vi "Dashboard Main.vi"() -> ()   [LabVIEW 2017]
uses:
  <vilib>/Rock Robotics/WPI/DriverStation/WPI_DriverStationAllianceInfo.ctl
  <vilib>/Rock Robotics/WPI/DriverStation/WPI_DriverStationPositionInfo.ctl
  <vilib>/Utility/miscctls.llb/LVRowAndColumnTypeDef.ctl
  <vilib>/event_ctls.llb/eventvkey.ctl
  <vilib>/Rock Robotics/Network Tables/NT Read Numeric Array.vi
  <vilib>/Rock Robotics/Network Tables/NT Write String Array.vi
  <vilib>/Rock Robotics/Network Tables/NT Write Numeric Array.vi
  <vilib>/Rock Robotics/Network Tables/NT Write Boolean.vi
  <vilib>/Rock Robotics/WPI/Dashboard/WPI_DashboardLogging Global.vi
panel:
  in  "Camera Settings Right":T1={"Frame Rate"=30, "Compression"=30, "Size"=1, "DB Camera Config"=FALSE} {"Frame Rate" scale=1.0..30.0; "Compression" scale=100.0..-1.0; "Size" items=["640x480", "320x240", "160x120"]}
  in  "Camera Name Right":string(combo)="No Camera Selection"
  out "Camera Info":cluster{"Mbps LED":bool, "Mbps":dbl, "fps":dbl} {"fps" format="%#.1g"; "Mbps" format="%#.1g"}
  in  "Camera Settings":T1={"Frame Rate"=30, "Compression"=30, "Size"=1, "DB Camera Config"=FALSE} {"Frame Rate" scale=1.0..30.0; "Compression" scale=100.0..-1.0; "Size" items=["640x480", "320x240", "160x120"]}
  in  "TCP":refnum<k5>
  in  "Rec Mode":enum32{"Stop", "Record", "Playback"}(radio)
  out "Robot IP":string
  out "Image Message":string="Timeout in Camera Communications"
  in  "Dashboard Tab":T2(tab)
  in  "Scooter Scale":dbl(slide)=0.49999999999999994 scale=0.0..1.0
  in  "Select Auto":string(combo)="Select Autonomous ..."
  out "NT Connection":bool
  out "MotorChart R":cluster{"Numeric":dbl, "Numeric":dbl}(graph)
  out "MotorChart L":cluster{"Numeric":dbl, "Numeric":dbl}(graph)
  out "MotorSliders R":cluster{"MotorSlide1":dbl, "MotorSlide2":dbl} {"MotorSlide2" scale=-1.0..1.0 scale format="%#_2e"; "MotorSlide1" scale=-1.0..1.0 scale format="%#_2e"}
  out "MotorSliders L":cluster{"MotorSlide1":dbl, "MotorSlide2":dbl} {"MotorSlide2" scale=-1.0..1.0 scale format="%#_2e"; "MotorSlide1" scale=-1.0..1.0 scale format="%#_2e"}
  out "Gyro":dbl(knob) scale=0.0..360.0
  out "JS1 Z":dbl(slide) scale=-1.0..1.0 scale format="%#_2e"
  out "JS1 Graph":cluster{"X":dbl, "Y":dbl}[](graph)
  out "JS1 Buttons":T3
  out "JS2 Z":dbl(slide) scale=-1.0..1.0 scale format="%#_2e"
  out "JS2 Graph":cluster{"X":dbl, "Y":dbl}[](graph)
  out "JS2 Buttons":T3
  out "Mode":T4(ring)=enum."Auto Disabled"
  out "Vision Angle":dbl
  out "Robot IP 2":string
  in  "Scooter Button":bool
  in  "Invert Drive?":bool
  out "Camera Image Right":T5(plugin-control)
  in  "DB/String 9":string
  in  "DB/String 8":string
  in  "DB/String 7":string
  in  "DB/String 6":string
  in  "DB/String 5":string
  in  "DB/String 4":string
  in  "DB/String 3":string
  in  "DB/String 2":string
  in  "DB/String 1":string
  in  "DB/String 0":string
  in  "DB/Slider 0":dbl(slide) scale=0.0..5.0
  in  "DB/Slider 1":dbl(slide) scale=0.0..5.0
  in  "DB/Slider 2":dbl(slide) scale=0.0..5.0
  in  "DB/Slider 3":dbl(slide) scale=0.0..5.0
  out "DB/LED 3":bool
  out "DB/LED 2":bool
  out "DB/LED 1":bool
  out "DB/LED 0":bool
  in  "DB/Button 3":bool
  in  "DB/Button 2":bool
  in  "DB/Button 1":bool
  in  "DB/Button 0":bool caption="New Name"
  out "Motor Outputs":T6 {"Motor 7" scale=-1.0..1.0; "Motor 6" scale=-1.0..1.0; "Motor 5" scale=-1.0..1.0; "Motor 4" scale=-1.0..1.0; "Motor 3" scale=-1.0..1.0; "Motor 2" scale=-1.0..1.0; "Motor 1" scale=-1.0..1.0; "Motor 0" scale=-1.0..1.0}
  out "Encoder Data":dbl[](array[numeric])
  out "NavX Data":dbl[](array[numeric])
  in  "Test Slider":dbl(slide) scale=0.0..100.0 scale format="%#_3g"
  in  "On/Off":bool caption="Solenoid"
  in  "Test Name":u16(ring) items=["Select the test to run..."]
  in  "Test Tree":string(tree)
  in  "Motor":cluster{"Value":dbl, "Enable":bool} {"Value" scale=-1.0..1.0 scale format="%#_3g"}
  out "Progress":T7 {"Test Progress" scale=0.0..100.0}
  in  "Rev/Fwd":cluster{"Forward":bool, "Reverse":bool}
  in  "Test Ring":u16(ring) items=["Monochrome", "Color"]
  out "Cmd Status":string
  in  "Execute Command":bool
  in  "Command Params":string[][](table)
  in  "Command Selection":i32(listbox)
  in  "CheckList":i32(listbox)
  out "Tree":string(tree)
  in  "Debug Data 2":dbl[](array[numeric])
  in  "Vision Target Offset":dbl=2.5
  in  "Vision Target Angle":dbl=15.0
  in  "Jog Mode Refnum":string(combo)="frontLeftRotation"
  out "Match Time":dbl
  in  "Debug Data":dbl[](array[numeric])
  in  "Debug Commands":string[](array[combo])
  in  "Debug Command?":bool
  out "Command Data":dbl[](array[numeric])
  out "Output Commands":string[](array[string])
  out "30 Amp Plugs":dbl[](array[slide]) scale=0.0..30.0
  out "40 Amp Plugs":dbl[](array[slide]) scale=0.0..40.0
  out "Ultrasonic Distance":dbl
  in  "Shooter Speed":dbl=0.575
  in  "Alliance":T8
  in  "Position":T9
  out "Command Data 2":dbl[](array[numeric])
  out "Camera Image":T5(plugin-control)
  out "Background":bool
  in  "Camera Name":string(combo)="No Camera Selection"
  # "HW"
  # "HW"
  # "Joysticks"
  # "Joystick 0 Layout\nAlign Left Gear: X\nAlign Middle Gear: A\nAlign Right Gear: B\nDrive To Shot Dist: Y\nVision Align: Left Bumper\nGear Place: Right Bumper\nBack: Command Stop\nStart: Reset Gyro\nR3: Jog Mode (Axis 1)\n\nJoystick 1 Layout\nShooter Forwards: Y\nShooter Backwards: A\nLift Up: B\nLift Down: Start\nLift Override Up: Back\nIntake In: Left Bumper\nIntake Out: Right Bumper\nAgitator In: D-Pad Up\nAgitator Out: D-Pad Down"
  # "Drive Motors"
  # "Front"
  # "Right"
  # "Left"
  # "Back"
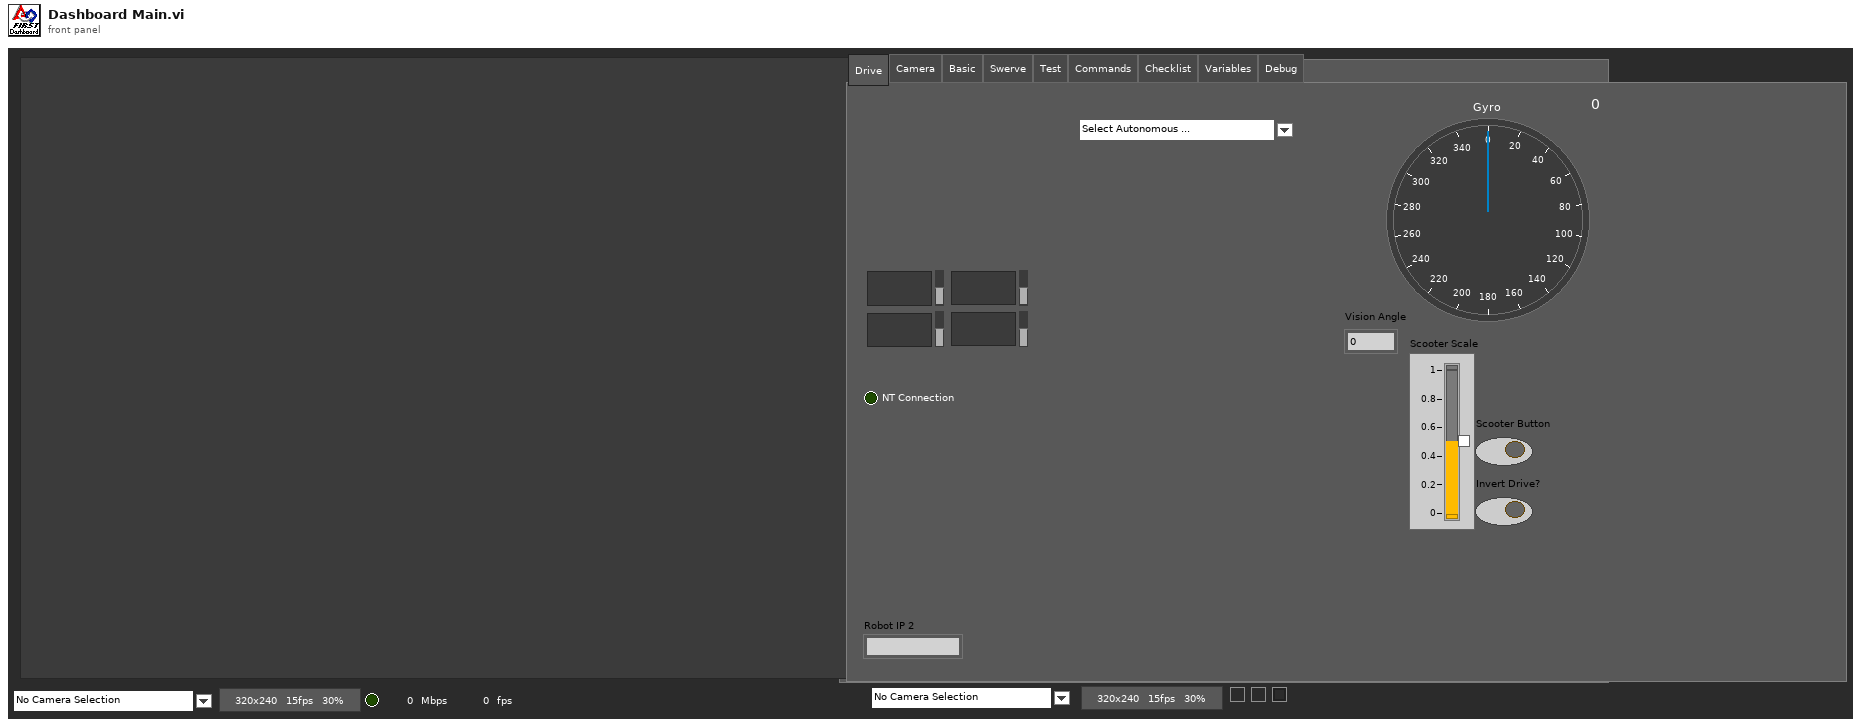
[diagram p1: front panel]
types:
  T1 = cluster{"Frame Rate":i32, "Compression":i32, "Size":u16, "DB Camera Config":bool}
  T2 = enum32{"Drive", "Camera", "Basic", "Swerve", "Test", "Commands", "Checklist", "Variables", "Debug"}
  T3 = cluster{bool, bool, bool, bool, bool, bool, bool, bool, bool, bool, bool, bool}
  T4 = enum8{"Tele-Op Disabled", "Tele-Op Enabled", "Auto Disabled", "Auto Enabled", "Test Disabled", "Test Enabled", "Disconnected", "No Code", "E-Stop"}
  T5 = typedef "IMAQ Image.ctl" = refnum<image>
  T6 = cluster{"Motor 0":dbl, "Motor 1":dbl, "Motor 2":dbl, "Motor 3":dbl, "Motor 4":dbl, "Motor 5":dbl, "Motor 6":dbl, "Motor 7":dbl}
  T7 = cluster{"Test Progress":u8, "Test Progress Text":string}
  T8 = typedef "WPI_DriverStationAllianceInfo.ctl" = enum16{"Red", "Blue", "Invalid"}
  T9 = typedef "WPI_DriverStationPositionInfo.ctl" = enum16{"1", "2", "3"}
  T10 = typedef "Image Type" = u32
  T11 = cluster{"IDs":cluster{"RPC field ID":u16, "Unique ID":u16}, "String":string}
  T12 = enum32{"Drive", "Basic", "Custom", "Test", "Checklist", "Variables"}
  T13 = cluster{"Camera Image":refnum<vi>, "Dashboard Tab":refnum<vi>, "Background":refnum<vi>, "Rec Mode":refnum<vi>, "Test Slider":refnum<vi>, "On/Off ":refnum<vi>, "Test Ring":refnum<vi>, "Rev/Fwd":refnum<vi>, "Test Name":refnum<vi>, "Motor":refnum<vi>, "Progress":refnum<vi>, "CheckList":refnum<vi>, "Tree":refnum<vi>, "Test Tree":refnum<vi>, "Command Params":refnum<vi>, "Command Selection":refnum<vi>, "Execute Command":refnum<vi>, "Cmd Status":refnum<vi>, "Camera Settings":refnum<vi>, "Camera Name":refnum<vi>, "Camera Info":refnum<vi>, "Camera Settings Right":refnum<vi>, "Camera Name Right":refnum<vi>, "Camera Image Right":refnum<vi>}
  T14 = enum8{"Enabled", "Disabled", "Disabled and Grayed Out"}
  T15 = cluster{"Error Strings":string, "Disable Counts":cluster{u16, u16}, "Rail Faults":cluster{u16, u16, u16}, "Robot IP":string, "DB Mode":u8, "Event Info":cluster{"Name":string, "Type":u8, "Number":u16, "Replay":u8}}
  T16 = cluster{"Storage":cluster{"Disk Free":u64, "RAM Block":u32, "RAM free":u32}, "CPU Utilization":cluster{"CPU % ISR":sgl, "CPU % Time Crit":sgl, "CPU % Timed Str":sgl, "CPU % High":sgl, "CPU % Above":sgl, "CPU % Normal":sgl, "CPU % Low":sgl}, "CAN":cluster{"% Bus Utilization":sgl, "Bus Off Cnt":u32, "TX_FIFO Full Cnt":u32, "Receive Error Cnt":u8, "Transmit Error Cnt":u8}, "HID":cluster{"HID Outputs":u32, "Rumble Low":u16, "Rumble High":u16}[]}
  T17 = cluster{"Status bits":cluster{"Test Mode":bool, "Autonomous":bool, "Enabled":bool, "Code Start":bool, "Brownout":bool, "Reserved 2":bool, "Reserved 3":bool, "E-Stop":bool}, "Code Trace":cluster{"Disabled":bool, "TeleOp":bool, "Auto":bool, "Test":bool}, "Controller Type":enum16{"unknown", "cRIO", "roboRio"}, "Code?":enum16{"unknown", "noCode", "code"}, "Battery V":dbl}
  T18 = cluster{"Control Bits":cluster{"TestMode":bool, "Autonomous":bool, "Enabled":bool, "FMS Present":bool, bool, bool, bool, "E-Stop":bool}, "Team Station ":u8, "Countdown":sgl, "Joystick Values":cluster{"Axes":dbl[], "Buttons":bool[], "POVs":i16[]}[]}
  T19 = cluster{"Axes":dbl[], "Buttons":bool[], "POVs":i16[]}[]
  T20 = cluster{"Numeric Array[0]":dbl, "Numeric Array[1]":dbl, "Numeric Array[2]":dbl, "Numeric Array[3]":dbl, "Numeric Array[4]":dbl, "Numeric Array[5]":dbl, "Numeric Array[6]":dbl, "Numeric Array[7]":dbl, "Numeric Array[8]":dbl}
  T21 = cluster{"Numeric Array[0]":dbl, "Numeric Array[1]":dbl, "Numeric Array[2]":dbl, "Numeric Array[3]":dbl, "Numeric Array[4]":dbl, "Numeric Array[5]":dbl, "Numeric Array[6]":dbl, "Numeric Array[7]":dbl}
  T22 = cluster{"Axes":dbl[], "Buttons":bool[], "POVs":i16[]}
  T23 = cluster{"Buttons[0]":bool, "Buttons[1]":bool, "Buttons[2]":bool, "Buttons[3]":bool, "Buttons[4]":bool, "Buttons[5]":bool, "Buttons[6]":bool, "Buttons[7]":bool, "Buttons[8]":bool, "Buttons[9]":bool, "Buttons[10]":bool, "Buttons[11]":bool}
  T24 = cluster{"Operation":enum16{"Update", "Clear"}, "Color Box":u32}[]
  T25 = typedef "eventvkey.ctl" = enum16{"ASCII", "Enter", "Return", "Shift", "Ctrl", "Alt", "Cmd", "Opt", "Caps", "NumLock", "Clear", "Break", "Up", "Down", "Left", "Right", "Insert", "Delete", "Home", "End", "PageUp", "PageDown", "Escape", "Help", "Pause", "ScrollLock", "F1", "F2", "F3", "F4", "F5", "F6", "F7", "F8", "F9", "F10", "F11", "F12", "F13", "F14", "F15", "F16", "F17", "F18", "F19", "F20", "F21", "F22", "F23", "F24", "Play", "VolumeUp", "VolumeDown", "Mute", "Two Byte Char"}
  T26 = cluster{"Image Size":bool, "Image Type":bool, "Pixel Value":bool, "ROI Information":bool, "Zoom Factor":bool}
  T27 = cluster{"Operation":enum16{"Update", "Clear"}, "Color Box":u32}
  T28 = typedef "LVRowAndColumnTypeDef.ctl" = cluster{"Row":i32, "Column":i32}
  T29 = cluster{"Shift":bool, "Ctrl":bool, "Alt":bool, "Cmd":bool, "Opt":bool}
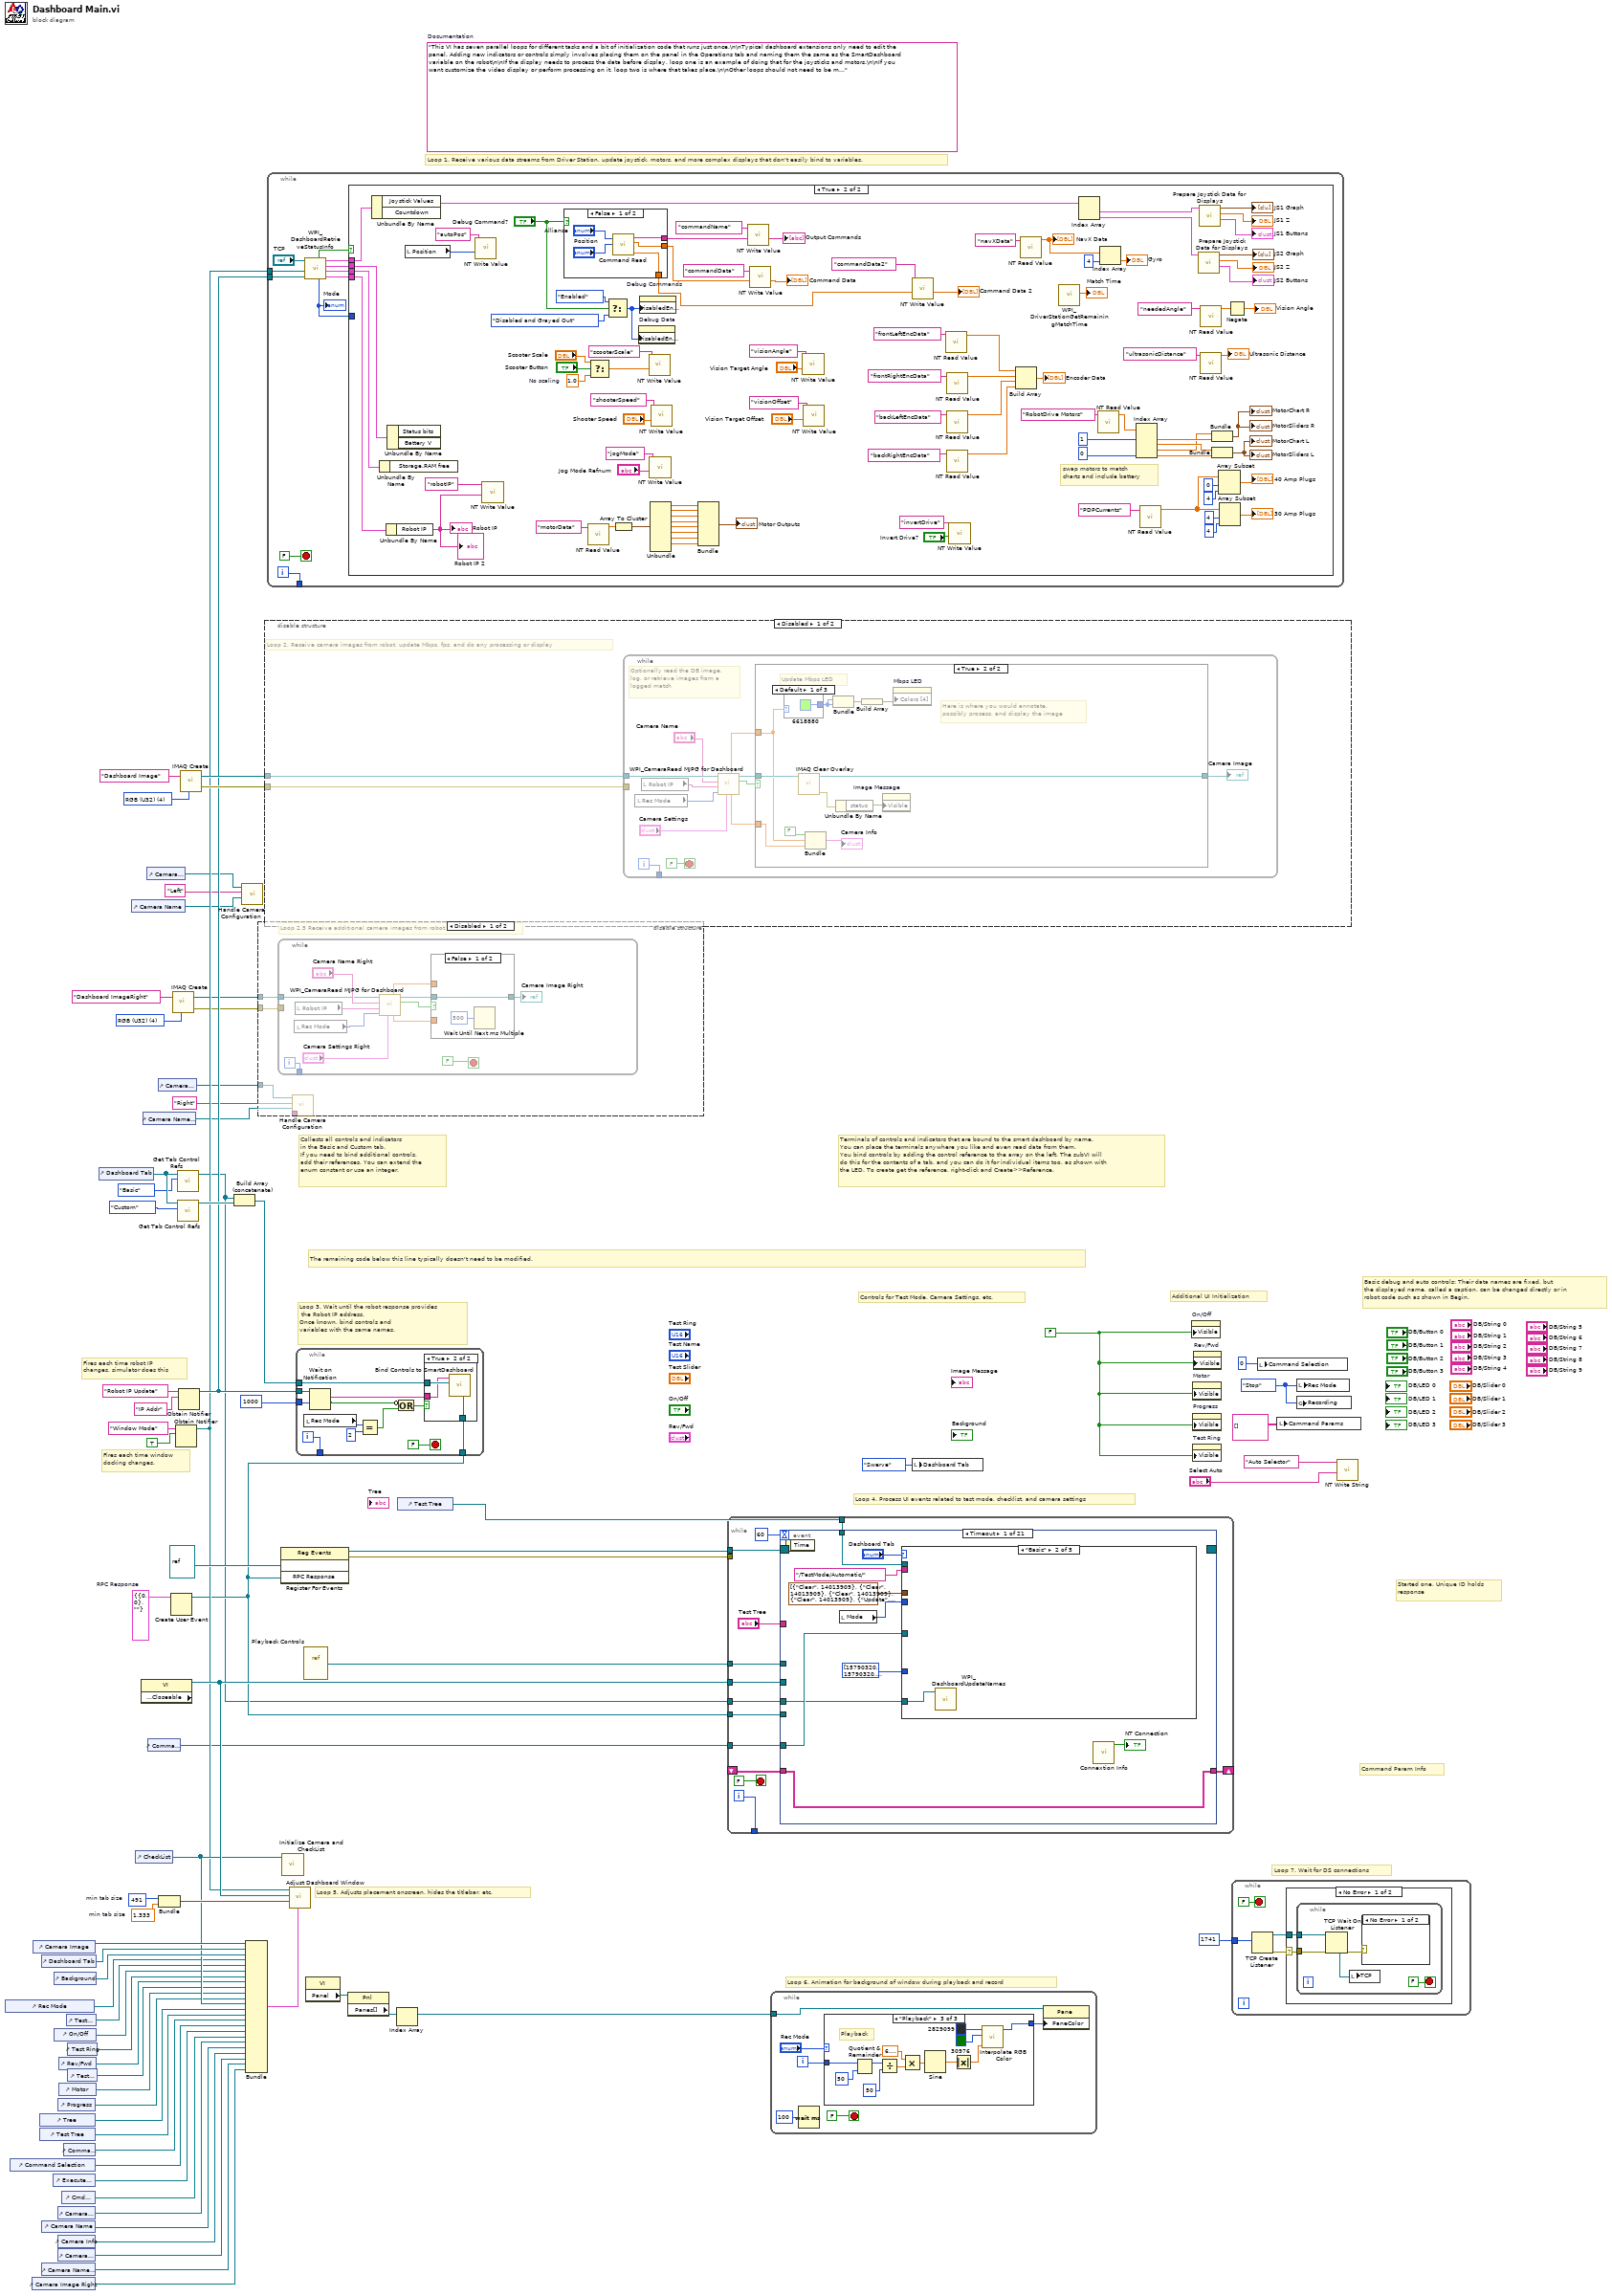
[diagram p0: block diagram]
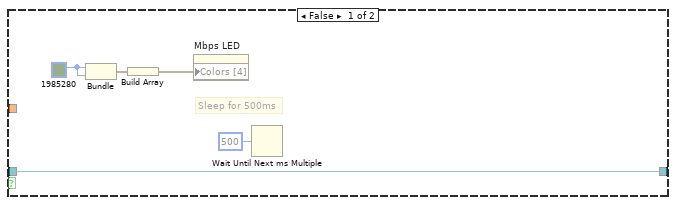
[diagram p2: hidden frame]
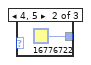
[diagram p3: hidden frame]
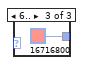
[diagram p4: hidden frame]
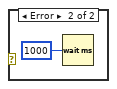
[diagram p8: hidden frame]
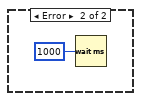
[diagram p9: hidden frame]
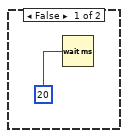
[diagram p10: hidden frame]
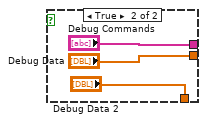
[diagram p11: hidden frame]
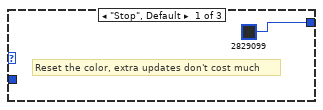
[diagram p12: hidden frame]
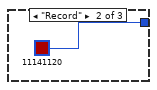
[diagram p13: hidden frame]
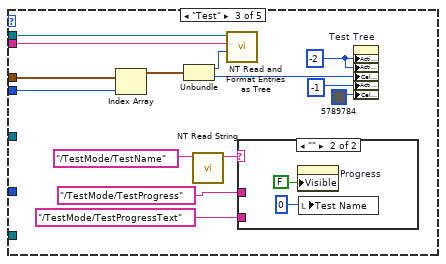
[diagram p16: hidden frame]
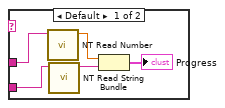
[diagram p17: hidden frame]
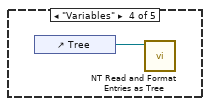
[diagram p18: hidden frame]
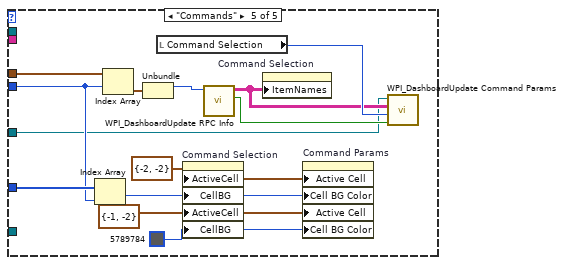
[diagram p19: hidden frame]
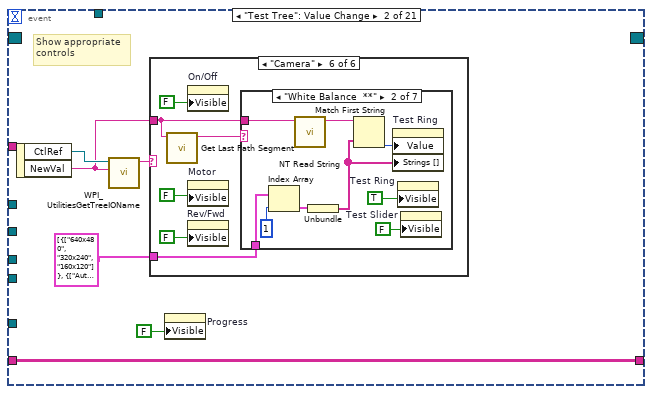
[diagram p20: hidden frame]
diagram:
  w11 = T10 4 items=["Grayscale (U8)", "Grayscale (I16)", "Grayscale (SGL)", "Complex (CSG)", "RGB (U32)", "HSL (U32)", "RGB (U64)"] ("Image Type")
  w27 = T11 {"IDs"={"RPC field ID"=0, "Unique ID"=0}, "String"=""}  # RPC Response
  w51 = 491  # min tab size
  w50 = 1.333  # min tab size
  w58 = enum32{"Stop", "Record", "Playback"}."Stop" ("Rec Mode")
  w33 = FALSE ("Visible")
  (unwired) "This VI has seven parallel loops for different tasks and a bit of initialization code that runs just once.\n\nTypical dashboard extensions only need to edit the panel. Adding new indicators or controls simply involves placing them on the panel in the Operations tab and naming them the same as the SmartDashboard variable on the robot\n\nIf the display needs to process the data before display, loop one is an example of doing that for the joysticks and motors.\n\nIf you want customize the video display or perform processing on it, loop two is where that takes place.\n\nOther loops should not need to be modified. They are pretty standard, and document the task they perform."  # Documentation
  w75 = T10 4 items=["Grayscale (U8)", "Grayscale (I16)", "Grayscale (SGL)", "Complex (CSG)", "RGB (U32)", "HSL (U32)", "RGB (U64)"] ("Image Type")
  # "Command Param Info"
  # "Started one, Unique ID holds\nresponse"
  # "Loop 7. Wait for DS connections"
  # "Basic debug and auto controls: Their data names are fixed, but\nthe displayed name, called a caption, can be changed directly or in\nrobot code such as shown in Begin."
  # "Controls for Test Mode, Camera Settings, etc."
  # "Additional UI Initialization"
  # "Loop 6. Animation for background of window during playback and record"
  # "Fires each time robot IP\nchanges, simulator does this"
  # "Fires each time window\ndocking changes."
  # "Collects all controls and indicators\nin the Basic and Custom tab.\nIf you need to bind additional controls,\nadd their references. You can extend the\nenum constant or use an integer."
  # "The remaining code below this line typically doesn't need to be modified."
  # "Loop 4. Process UI events related to test mode, checklist, and camera settings"
  # "Terminals of controls and indicators that are bound to the smart dashboard by name.\nYou can place the terminals anywhere you like and even read data from them.\nYou bind controls by adding the control reference to the array on the left. The subVI will\ndo this for the contents of a tab, and you can do it for individual items too, as shown with\nthe LED. To create get the reference, right-click and Create>>Reference."
  # "Loop 3. Wait until the robot response provides\n the Robot IP address.\nOnce known, bind controls and\nvariables with the same names."
  # "Loop 5. Adjusts placement onscreen, hides the titlebar, etc."
  # "Loop 1. Receive various data streams from Driver Station, update joystick, motors, and more complex displays that don't easily bind to variables."
  n1 = control-ref of="Rec Mode"() -> (w39:refnum<vi>)
  n2 = control-ref of="Command Selection"() -> (w26:refnum<vi>)
  n3 = control-ref of="Camera Image Right"() -> (w2:refnum<vi>)
  n4 = control-ref of="Camera Image"() -> (w53:refnum<vi>)
  n5 = control-ref of="Tree"() -> (w43:refnum<vi>)
  n6 = control-ref of="Test Tree"() -> (w42:refnum<vi>)
  n7 = control-ref of="Dashboard Tab"() -> (w52:refnum<vi>)
  n8 = control-ref of="Camera Name"() -> (w17:refnum<vi>)
  n9 = control-ref of="Camera Name Right"() -> (w3:refnum<vi>)
  n10 = control-ref of="Execute Command"() -> (w28:refnum<vi>)
  n11 = control-ref of="Background"() -> (w48:refnum<vi>)
  n12 = control-ref of="On/Off"() -> (w37:refnum<vi>)
  n13 = control-ref of="Progress"() -> (w34:refnum<vi>)
  n14 = control-ref of="Camera Settings"() -> (w18:refnum<vi>)
  n15 = control-ref of="Camera Info"() -> (w16:refnum<vi>)
  n16 = control-ref of="Camera Settings Right"() -> (w4:refnum<vi>)
  n17 = control-ref of="Rev/Fwd"() -> (w35:refnum<vi>)
  n18 = control-ref of="Motor"() -> (w40:refnum<vi>)
  n19 = control-ref of="Cmd Status"() -> (w22:refnum<vi>)
  n20 = control-ref of="Command Params"() -> (w29:refnum<vi>)
  n21 = control-ref of="Test Slider"() -> (w38:refnum<vi>)
  n22 = control-ref of="Test Ring"() -> (w36:refnum<vi>)
  n23 = control-ref of="Test Name"() -> (w41:refnum<vi>)
  n24 = control-ref of="Dashboard Tab"() -> (w56:refnum<vi>)
  n25 = control-ref of="Camera Name"() -> (w19:refnum<vi>)
  n26 = control-ref of="CheckList"() -> (w44:refnum<vi>)
  n27 = property class="VI" props=["Front Panel.Closeable"]() -> (reference out=w57:refnum<vi>)  [unwired: 2 in, 2 out]
  n28 = control-ref of="Camera Name Right"() -> (w7:refnum<vi>)
  n29 = control-ref of="Camera Settings"() -> (w20:refnum<vi>)
  n30 = control-ref of="Command Params"() -> (w21:refnum<vi>)
  n31 = control-ref of="Camera Settings Right"() -> (w8:refnum<vi>)
  n32 = Bundle("min tab size"=w51, "min tab size"=w50) -> (w49:cluster{"min tab size":i32, "min tab size":dbl})  [unwired: 1 in]
  n33 = Create User Event(user event datatype=w27) -> (user event=w23:refnum<user-event>)  [unwired: 1 in, 1 out]
  n34 = call "IMAQ Create"("Image Name"="Dashboard ImageRight", "Image Type"=w11) -> ("New Image"=w10:T5, "error out"=w9:errorcluster)  [unwired: 2 in, 1 out]
  n35 = Obtain Notifier(name (unnamed)="Window Mode", notification data type=TRUE) -> (notifier out=w31:refnum<notifier>)  [unwired: 2 in, 2 out]
  n36 = call <vilib>:"Get Tab Control Refs.vi"("Page Index"=T12."Basic" ("Dashboard Tab"), "TabControl in"=w56) -> ("ControlsOnPage"=w15:refnum<vi>[])  [unwired: 9 in]
  n37 = call <vilib>:"Get Tab Control Refs.vi"("Page Index"=T12."Custom" ("Dashboard Tab"), "TabControl in"=w56) -> ("ControlsOnPage"=w55:refnum<vi>[])  [unwired: 9 in]
  n38 = Obtain Notifier(name (unnamed)="Robot IP Update", notification data type="IP Addr" ("name (unnamed)")) -> (notifier out=w32:refnum<notifier>)  [unwired: 2 in, 2 out]
  n39 = call "IMAQ Create"("Image Name"="Dashboard Image", "Image Type"=w75) -> ("New Image"=w73:T5, "error out"=w72:errorcluster)  [unwired: 2 in, 1 out]
  n40 = Build Array (concatenate)(w15, w55) -> (w54:refnum<vi>[])
  n41 = call "Handle Camera Configuration.vi"("CameraNameRef"=w19, "Camera File Name"="Left", "ClusterRef"=w20) -> ()  [unwired: 9 in]
  n42 = Bundle("Camera Image"=w53, "Dashboard Tab"=w52, "Background"=w48, "Rec Mode"=w39, "Test Slider"=w38, "On/Off"=w37, "Test Ring"=w36, "Rev/Fwd"=w35, "Test Name"=w41, "Motor"=w40, "Progress"=w34, "CheckList"=w44, "Tree"=w43, "Test Tree"=w42, "Command Params"=w29, "Command Selection"=w26, "Execute Command"=w28, "Cmd Status"=w22, "Camera Settings"=w18, "Camera Name"=w17, "Camera Info"=w16, "Camera Settings Right"=w4, "Camera Name Right"=w3, "Camera Image Right"=w2) -> (w45:T13)  [unwired: 1 in]
  n43 = disable-structure shown="Disabled" {
    disable-tunnel: w10 -> [w80 _]
    disable-tunnel: w9 -> [w79 _]
    disable-tunnel: w8 -> [w78 _]
    disable-tunnel: w7 -> [w77 _]
    disable-tunnel: "Right" -> [w76 _]
    frame Disabled {
      # "Loop 2.5 Receive additional camera images from robot and display"
      n44 = while {
        tunnel: w80 -> [w91]
        tunnel: w79 -> [_]
        tunnel: [w85] -> _
        i -> [w85]
        stop <- FALSE stop-if-true
        n45 = local read "Rec Mode"() -> (w89:enum32{"Stop", "Record", "Playback"})
        n46 = local read "Robot IP"() -> (w90:string)
        n47 = call <vilib>:"WPI_CameraRead MJPG for Dashboard.vi"("Camera Settings"="Camera Settings Right", "Rec Mode"=w89, "NT Connection"=w90, "Capture Info"="Camera Name Right", "Refnum in"=w91) -> ("Active"=w84:bool, "Refnum out"=w87:T5, "FPS"=w82:dbl, "Bandwidth (Mbps)"=w83:dbl)  [unwired: 3 in]
        n48 = case shown="False" w84 {
          tunnel: w87 -> [w93 w95]
          tunnel: w83 -> [_ _]
          tunnel: w82 -> [_ _]
          tunnel: [w93 w95] -> w81
          frame False {
            n49 = Wait Until Next ms Multiple(millisecond multiple=u32 500) -> ()  [unwired: 1 out]
          }
          frame True {
          }
        }
        "Camera Image Right" <- w81
      }
      n50 = call "Handle Camera Configuration.vi"("CameraNameRef"=w77, "Camera File Name"=w76, "ClusterRef"=w78) -> ()  [unwired: 9 in]
    }
    frame Enabled {
    }
  }
  n51 = disable-structure shown="Disabled" {
    disable-tunnel: w73 -> [w97 _]
    disable-tunnel: w72 -> [w96 _]
    frame Disabled {
      # "Loop 2. Receive camera images from robot, update Mbps, fps, and do any processing or display"
      n52 = while {
        tunnel: w97 -> [w107]
        tunnel: w96 -> [_]
        tunnel: [w108] -> _
        i -> [w108]
        stop <- FALSE stop-if-true
        # "Optionally read the DB image,\nlog, or retrieve images from a\nlogged match"
        n53 = local read "Rec Mode"() -> (w103:enum32{"Stop", "Record", "Playback"})
        n54 = local read "Robot IP"() -> (w102:string)
        n55 = call <vilib>:"WPI_CameraRead MJPG for Dashboard.vi"("Camera Settings"="Camera Settings", "Rec Mode"=w103, "NT Connection"=w102, "Capture Info"="Camera Name", "Refnum in"=w107) -> ("Active"=w105:bool, "Refnum out"=w106:T5, "FPS"=w104:dbl, "Bandwidth (Mbps)"=w101:dbl)  [unwired: 3 in]
        n56 = case shown="True" w105 {
          tunnel: w106 -> [w110 w121]
          tunnel: w101 -> [_ w118]
          tunnel: w104 -> [_ w119]
          tunnel: [w110 w115] -> w98
          frame False {
            w112 = u32 1985280 ("Color Box")
            # "Sleep for 500ms"
            n57 = Bundle("Color Box"=w112, "Color Box"=w112) -> (w113:cluster{"Color Box":u32, "Color Box":u32})  [unwired: 1 out]
            n58 = Build Array(w113) -> (w111:cluster{"Color Box":u32, "Color Box":u32}[])
            n59 = property on="Mbps LED" class="Bool (strict)"("Colors [4]"=w111) -> ()  [unwired: 2 in, 2 out]
            n60 = Wait Until Next ms Multiple(millisecond multiple=u32 500) -> ()  [unwired: 1 out]
          }
          frame True {
            # "Here is where you would annotate,\npossibly process, and display the image"
            # "Update Mbps LED"
            n61 = case shown="Default" w118 {
              tunnel: [u32 6618880 ("Color Box") u32 16776722 ("Color Box") u32 16716800 ("Color Box")] -> w122
              frame Default {
              }
              frame 4, 5 {
              }
              frame 6.. {
              }
            }
            n62 = call "IMAQ Clear Overlay"("Image"=w121) -> ("error out"=w124:errorcluster, "Image Out"=w115:T5)  [unwired: 2 in, 7 out]
            n63 = Bundle(FALSE, "Bandwidth (Mbps)"=w118, "FPS"=w119) -> (→"Camera Info":cluster{bool, "Bandwidth (Mbps)":dbl, "FPS":dbl})  [unwired: 1 in]
            n64 = Bundle("Color Box"=w122, "Color Box"=w122) -> (w123:cluster{"Color Box":u32, "Color Box":u32})  [unwired: 1 out]
            n65 = Unbundle By Name(w124) -> ("status"=w125:bool)
            n66 = Build Array(w123) -> (w120:cluster{"Color Box":u32, "Color Box":u32}[])
            n67 = property on="Image Message" class="Str"("Visible"=w125) -> ()  [unwired: 2 in, 2 out]
            n68 = property on="Mbps LED" class="Bool (strict)"("Colors [4]"=w120) -> ()  [unwired: 2 in, 2 out]
          }
        }
        "Camera Image" <- w98
      }
    }
    frame Enabled {
    }
  }
  n69 = while {
    tunnel: [w138] -> _
    tunnel: w32 -> [w132]
    tunnel: w31 -> [w129]
    i -> [w138]
    stop <- FALSE stop-if-true
    n70 = call <vilib>:"WPI_DashboardRetrieveStatusInfo.vi"("Binding Refnum"=w132, "Window Mode Notifier"=w129, "TCP Cnx"="TCP") -> ("Power and Errors"=w133:T15, "Robot Metrics"=w136:T16, "Status Info"=w137:T17, "Control Info"=w134:T18, "Robot Mode"=w131:T4, "Process?"=w135:bool)  [unwired: 3 in]
    "Mode" <- w131
    n71 = case shown="True" w135 {
      tunnel: w137 -> [_ w231]
      tunnel: w136 -> [_ w230]
      tunnel: w134 -> [_ w229]
      tunnel: w133 -> [_ w228]
      tunnel: w131 -> [_ _]
      frame False {
        n72 = Wait (ms)(milliseconds to wait=u32 20) -> ()  [unwired: 1 out]
      }
      frame True {
        w173 = 1.0  # No scaling
        # "swap motors to match\ncharts and include battery"
        n73 = Unbundle By Name(w229) -> ("Joystick Values"=w219:T19)  [unwired: 1 out]
        n74 = Unbundle By Name(w230) -> ()  [unwired: 1 out]
        n75 = Unbundle By Name(w228) -> ("Robot IP"=w168:string)
        "Robot IP" <- w168
        "Robot IP 2" <- w168
        n76 = Unbundle By Name(w231) -> ()  [unwired: 2 out]
        n77 = local read "Position"() -> (w145:T9)
        n78 = call-poly <vilib>:"NT Write Value.vi"("Numeric"=w145, "Name"="autoPos") -> ()  [unwired: 9 in, 1 out]
        n79 = call-poly <vilib>:"NT Write Value.vi"("String"=w168, "Name"="robotIP") -> ()  [unwired: 9 in, 1 out]
        n80 = case shown="False" "Debug Command?" {
          tunnel: [w233 "Debug Data"] -> w164
          tunnel: [w234 "Debug Commands"] -> w163
          tunnel: [w232 "Debug Data 2"] -> w141
          frame False {
            n81 = call "Command Read.vi"("Position"="Position", "Alliance"="Alliance") -> ("value 2"=w232:dbl[], "value"=w233:dbl[], "command"=w234:string[])  [unwired: 5 in, 1 out]
          }
          frame True {
          }
        }
        "Output Commands" <- w163
        "Command Data" <- w164
        "Command Data 2" <- w141
        n82 = call-poly <vilib>:"NT Read Value.vi"("Name"="motorData") -> ("Numeric Array"=w197:dbl[])  [unwired: 9 in, 1 out]
        n83 = Select(t="Scooter Scale", s="Scooter Button", f=w173) -> (s? t:f=w172:dbl)
        n84 = Select(t=T14."Enabled" ("Disabled"), s="Debug Command?", f=T14."Disabled and Grayed Out" ("Disabled")) -> (s? t:f=w156:T14)
        n85 = Array To Cluster(array=w197) -> (cluster=w196:T20)
        n86 = property on="Debug Data" class="Arr (strict)"("DisabledEnum"=w156) -> ()  [unwired: 2 in, 2 out]
        n87 = property on="Debug Commands" class="Arr (strict)"("DisabledEnum"=w156) -> ()  [unwired: 2 in, 2 out]
        n88 = call-poly <vilib>:"NT Write Value.vi"("Numeric"=w172, "Name"="scooterScale") -> ()  [unwired: 9 in, 1 out]
        n89 = call-poly <vilib>:"NT Write Value.vi"("String"="Jog Mode Refnum", "Name"="jogMode") -> ()  [unwired: 9 in, 1 out]
        n90 = Unbundle(w196) -> ("Numeric Array[0]"=w195:dbl, "Numeric Array[1]"=w194:dbl, "Numeric Array[2]"=w193:dbl, "Numeric Array[3]"=w192:dbl, "Numeric Array[4]"=w191:dbl, "Numeric Array[5]"=w190:dbl, "Numeric Array[6]"=w189:dbl, "Numeric Array[7]"=w188:dbl)  [unwired: 1 out]
        n91 = call-poly <vilib>:"NT Write Value.vi"("Numeric"="Shooter Speed", "Name"="shooterSpeed") -> ()  [unwired: 9 in, 1 out]
        n92 = Bundle("Numeric Array[0]"=w195, "Numeric Array[1]"=w194, "Numeric Array[2]"=w193, "Numeric Array[3]"=w192, "Numeric Array[4]"=w191, "Numeric Array[5]"=w190, "Numeric Array[6]"=w189, "Numeric Array[7]"=w188) -> (→"Motor Outputs":T21)  [unwired: 1 in]
        n93 = call-poly <vilib>:"NT Write Value.vi"("String Array"=w163, "Name"="commandName") -> ()  [unwired: 9 in, 1 out]
        n94 = call-poly <vilib>:"NT Write Value.vi"("Numeric Array"=w164, "Name"="commandData") -> ()  [unwired: 9 in, 1 out]
        n95 = call-poly <vilib>:"NT Write Value.vi"("Numeric"="Vision Target Angle", "Name"="visionAngle") -> ()  [unwired: 9 in, 1 out]
        n96 = call-poly <vilib>:"NT Write Value.vi"("Numeric"="Vision Target Offset", "Name"="visionOffset") -> ()  [unwired: 9 in, 1 out]
        n97 = call-poly <vilib>:"NT Write Value.vi"("Numeric Array"=w141, "Name"="commandData2") -> ()  [unwired: 9 in, 1 out]
        n98 = call-poly <vilib>:"NT Read Value.vi"("Name"="frontLeftEncData") -> ("Numeric"=w203:dbl)  [unwired: 9 in, 1 out]
        n99 = call-poly <vilib>:"NT Read Value.vi"("Name"="frontRightEncData") -> ("Numeric"=w202:dbl)  [unwired: 9 in, 1 out]
        n100 = call-poly <vilib>:"NT Read Value.vi"("Name"="backLeftEncData") -> ("Numeric"=w201:dbl)  [unwired: 9 in, 1 out]
        n101 = call-poly <vilib>:"NT Read Value.vi"("Name"="backRightEncData") -> ("Numeric"=w200:dbl)  [unwired: 9 in, 1 out]
        n102 = call-poly <vilib>:"NT Write Value.vi"("Boolean"="Invert Drive?", "Name"="invertDrive") -> ()  [unwired: 9 in, 1 out]
        n103 = Build Array(w203, w202, w201, w200) -> (→"Encoder Data":dbl[])
        n104 = call-poly <vilib>:"NT Read Value.vi"("Name"="navXData") -> ("Numeric Array"=w186:dbl[])  [unwired: 9 in, 1 out]
        "NavX Data" <- w186
        n105 = call <vilib>:"WPI_DriverStationGetRemainingMatchTime.vi"() -> ("Match Time(s)"=→"Match Time":sgl)  [unwired: 10 in, 1 out]
        n106 = Index Array(array=w219) -> (element #1=w218:T22, element #2=w214:T22)  [unwired: 2 in]
        n107 = call-poly <vilib>:"NT Read Value.vi"("Name"="RobotDrive Motors") -> ("Numeric Array"=w209:dbl[])  [unwired: 9 in, 1 out]
        n108 = Index Array(array=w186, index=4) -> (element=→"Gyro":dbl)
        n109 = Index Array(array=w209, index #1=1, index #4=0) -> (element #1=w223:dbl, element #2=w224:dbl, element #3=w222:dbl, element #4=w227:dbl)  [unwired: 2 in]
        n110 = call-poly <vilib>:"NT Read Value.vi"("Name"="PDPCurrents") -> ("Numeric Array"=w180:dbl[])  [unwired: 9 in, 1 out]
        n111 = call "Prepare Joystick Data for Displays.vi"("Joystick Values"=w214) -> ("Buttons"=→"JS2 Buttons":T23, "Z Axis"=→"JS2 Z":dbl, "Cartesian Data"=→"JS2 Graph":cluster{"X axis":dbl, "X axis":dbl}[])  [unwired: 8 in]
        n112 = call "Prepare Joystick Data for Displays.vi"("Joystick Values"=w218) -> ("Buttons"=→"JS1 Buttons":T23, "Z Axis"=→"JS1 Z":dbl, "Cartesian Data"=→"JS1 Graph":cluster{"X axis":dbl, "X axis":dbl}[])  [unwired: 8 in]
        n113 = call-poly <vilib>:"NT Read Value.vi"("Name"="neededAngle") -> ("Numeric"=w152:dbl)  [unwired: 9 in, 1 out]
        n114 = call-poly <vilib>:"NT Read Value.vi"("Name"="ultrasonicDistance") -> ("Numeric"=→"Ultrasonic Distance":dbl)  [unwired: 9 in, 1 out]
        n115 = Bundle("Numeric"=w222, "Numeric"=w223) -> (→"MotorChart R" →"MotorSliders R":cluster{"Numeric":dbl, "Numeric":dbl})  [unwired: 1 in]
        n116 = Bundle("Numeric"=w224, "Numeric"=w227) -> (→"MotorChart L" →"MotorSliders L":cluster{"Numeric":dbl, "Numeric":dbl})  [unwired: 1 in]
        n117 = Array Subset(array=w180, index=0, length=4) -> (→"40 Amp Plugs":dbl[])
        n118 = Array Subset(array=w180, index=4, length=4) -> (→"30 Amp Plugs":dbl[])
        n119 = Negate(x=w152) -> (-x=→"Vision Angle":dbl)
      }
    }
  }
  n120 = register-events(refnum<vi> refnum, w23) -> (reference out=w62:refnum<event-registration>, error out=w61:errorcluster)  [unwired: 2 in]
  n121 = call "Initialize Camera and CheckList.vi"("ListBox in"=w44) -> ()  [unwired: 11 in]
  n122 = call "Adjust Dashboard Window.vi"("Sizing Refnums"=w45, "Size Constraints"=w49, "VI"=w57, "WIn Mode"=w31) -> ()  [unwired: 8 in]
  n123 = while {
    tunnel: w54 -> [w251]
    tunnel: w32 -> [w249]
    tunnel: [w247] -> _
    tunnel: u32 1000 ("milliseconds to wait") -> [w246]
    tunnel: w23 -> [w240]
    i -> [w247]
    stop <- FALSE stop-if-true
    n124 = local read "Rec Mode"() -> (w242:enum32{"Stop", "Record", "Playback"})
    n125 = Wait on Notification(notifier=w249, timeout in ms (-1)=w246) -> (notification=w248:string, timed out?=w244:bool)  [unwired: 2 in, 2 out]
    n126 = Equal?(x=w242, y=u16 2 ("Rec Mode")) -> (x = y?=w243:bool)
    n127 = Compound Arithmetic op=OR(invert w244, w243) -> (w245:bool)
    n128 = case shown="True" w245 {
      tunnel: w251 -> [_ w254]
      tunnel: w248 -> [_ w253]
      tunnel: w240 -> [_ w252]
      frame False {
      }
      frame True {
        n129 = call <vilib>:"Bind Controls to SmartDashboard.vi"("RPC ref"=w252, "Bound Control Refs"=w254, "Server IP Address"=w253) -> ()  [unwired: 9 in]
      }
    }
  }
  n130 = vi-ref "Playback Controls.vi"() -> (w63:refnum<vi>)
  n131 = property class="VI"() -> ("Panel"=w65:refnum<vi>)  [unwired: 2 in, 2 out]
  n132 = property class="Pnl"(reference=w65) -> ("Panes[]"=w66:refnum<vi>[])  [unwired: 1 in, 2 out]
  n133 = Index Array(array=w66) -> (element=w64:refnum<vi>)  [unwired: 1 in]
  n134 = control-ref of="Test Tree"() -> (w67:refnum<vi>)
  n135 = while {
    tunnel: [w264] -> _
    tunnel: w67 -> [w263]
    tunnel: w63 -> [w262]
    tunnel: w62 -> [w261]
    tunnel: w61 -> [_]
    tunnel: w57 -> [w260]
    tunnel: w23 -> [w259]
    tunnel: w21 -> [w258]
    shift-right: [w257] -> _
    shift-left: _ -> [w256]
    tunnel: w15 -> [w255]
    i -> [w264]
    stop <- FALSE stop-if-true
    n136 = event shown="[0] Timeout" {
      selector: w261 -> [_ _ _ _ _ _ _ _ _ _ _ _ _ _ _ _ _ _ _ _ _]
      dyn-events: [_ _ _ _ _ _ _ _ _ _ _ _ _ _ _ _ w520 _ _ _ _] -> _
      timeout: u32 60 ("milliseconds to wait") -> [_ _ _ _ _ _ _ _ _ _ _ _ _ _ _ _ _ _ _ _ _]
      tunnel: w263 -> [w276 _ _ _ _ _ _ _ _ _ _ _ _ _ _ _ _ _ _ _ _]
      tunnel: "Test Tree" -> [_ _ _ _ _ _ _ _ _ _ _ w487 w495 w497 w501 w509 _ _ _ _ _]
      tunnel: w262 -> [_ _ _ _ _ _ _ _ _ _ _ _ _ _ _ _ w522 _ w540 _ _]
      tunnel: w260 -> [_ _ _ _ _ _ _ _ _ _ _ _ _ _ _ _ w518 _ _ _ _]
      tunnel: w259 -> [_ _ _ _ _ _ _ _ _ _ _ _ _ _ _ _ w514 _ _ _ _]
      tunnel: w258 -> [w271 _ _ _ _ _ w438 _ _ _ _ _ _ _ _ _ _ _ _ _ _]
      tunnel: [w270 w315 w417 w422 w431 w435 w436 w445 w455 w462 w474 w486 w493 w496 w500 w508 w513 w535 w537 w541 w552] -> w257
      tunnel: w256 -> [w270 w315 w417 w422 w431 w435 w436 _ _ w462 w474 w486 w493 w496 w500 w508 w513 w535 w537 w541 w552]
      tunnel: w255 -> [w268 _ _ _ _ _ _ _ _ _ _ _ _ _ _ _ _ _ _ _ _]
      event Timeout {
        n137 = event-data() -> ()  [unwired: 1 in, 1 out]
        n138 = local read "Mode"() -> (w273:T4)
        n139 = case shown="\"Basic\"" "Dashboard Tab" {
          tunnel: w276 -> [_ _ w292 _ _]
          tunnel: "/TestMode/Automatic/" ("Name Pattern") -> [_ _ w291 _ _]
          tunnel: T24 [{"Operation"=enum."Clear", "Color Box"=14013909}, {"Operation"=enum."Clear", "Color Box"=14013909}, {"Operation"=enum."Clear", "Color Box"=14013909}, {"Operation"=enum."Clear", "Color Box"=14013909}, {"Operation"=enum."Update", "Color Box"=14013909}, {"Operation"=enum."Update", "Color Box"=16777215}, {"Operation"=enum."Clear", "Color Box"=14013909}, {"Operation"=enum."Clear", "Color Box"=14013909}, {"Operation"=enum."Clear", "Color Box"=14013909}] -> [_ _ w284 _ w308]
          tunnel: w273 -> [_ _ w283 _ w307]
          tunnel: u32[] [15790320, 15790320, 15790320, 15790320, 16777215, 16777215, 15790320, 15790320, 15790320] -> [_ _ _ _ w313]
          tunnel: w271 -> [_ _ _ _ w301]
          tunnel: w268 -> [_ w278 _ _ _]
          frame "Swerve", Default {
          }
          frame "Basic" {
            n140 = call <vilib>:"WPI_DashboardUpdateNames.vi"("Controls on Tab"=w278) -> ()  [unwired: 11 in]
          }
          frame "Test" {
            w290 = -2 ("Active Item:Row Number")
            n141 = Index Array(array=w284, index=w283) -> (element=w285:T27)
            n142 = Unbundle(w285) -> ("Operation"=w286:enum16{"Update", "Clear"}, "Color Box"=w287:u32)
            n143 = call <vilib>:"NT Read String.vi"("Name"="/TestMode/TestName") -> ("String"=w281:string)  [unwired: 9 in, 1 out]
            n144 = call <vilib>:"NT Read and Format Entries as Tree.vi"("Operation"=w286, "Name Pattern"=w291, "Tree Refnum"=w292) -> ()  [unwired: 7 in, 2 out]
            n145 = case shown="\"\"" w281 {
              tunnel: "/TestMode/TestProgress" ("Name") -> [w294 _]
              tunnel: "/TestMode/TestProgressText" ("Name") -> [w293 _]
              frame Default {
                n146 = call <vilib>:"NT Read Number.vi"("Name"=w294) -> ("Numeric"=w295:dbl)  [unwired: 9 in, 1 out]
                n147 = call <vilib>:"NT Read String.vi"("Name"=w293) -> ("String"=w296:string)  [unwired: 9 in, 1 out]
                n148 = Bundle("Numeric"=w295, "String"=w296) -> (→"Progress":cluster{"Numeric":dbl, "String":string})  [unwired: 1 in]
              }
              frame "" {
                n149 = property on="Progress" class="Clust (strict)"("Visible"=FALSE) -> ()  [unwired: 2 in, 2 out]
                n150 = local write "Test Name"(u16 0) -> ()
              }
            }
            n151 = property on="Test Tree" class="Tree (strict)"("Active Item Row Number"=w290, "ActiveColNum"=w290, "CellBG"=w287, "Active Item Row Number"=-1 ("Active Item:Row Number"), "CellBG"=u32 5789784 ("Color Box")) -> ()  [unwired: 2 in, 2 out]
          }
          frame "Variables" {
            n152 = control-ref of="Tree"() -> (w300:refnum<vi>)
            n153 = call <vilib>:"NT Read and Format Entries as Tree.vi"("Tree Refnum"=w300) -> ()  [unwired: 9 in, 2 out]
          }
          frame "Commands" {
            w309 = u32 5789784 ("Color Box")
            w310 = T28 {"Row"=-1, "Column"=-2} ("Active Cell:Active Cell")
            w312 = T28 {"Row"=-2, "Column"=-2} ("Active Cell:Active Cell")
            n154 = Index Array(array=w313, index=w307) -> (element=w311:u32)
            n155 = Index Array(array=w308, index=w307) -> (element=w306:T27)
            n156 = Unbundle(w306) -> ("Operation"=w305:enum16{"Update", "Clear"})  [unwired: 1 out]
            n157 = local read "Command Selection"() -> (w304:i32)
            n158 = property on="Command Selection" class="MCListbox (strict)"("ActiveCell"=w312, "CellBG"=w311, "ActiveCell"=w310, "CellBG"=w309) -> ()  [unwired: 2 in, 2 out]
            n159 = call <vilib>:"WPI_DashboardUpdate RPC Info.vi"("Operation"=w305) -> ("update"=w303:bool, "commands"=w302:string[][])  [unwired: 9 in]
            n160 = property on="Command Selection" class="MCListbox (strict)"("ItemNames"=w302) -> ()  [unwired: 2 in, 2 out]
            n161 = property on="Command Params" class="Tbl (strict)"("Active Cell"=w312, "Cell BG Color"=w311, "Active Cell"=w310, "Cell BG Color"=w309) -> ()  [unwired: 2 in, 2 out]
            n162 = call <vilib>:"WPI_DashboardUpdate Command Params.vi"("Update"=w303, "NewVal"=w304, "Commands"=w302, "Param Tbl"=w301) -> ()  [unwired: 7 in, 1 out]
          }
        }
        n163 = call <vilib>:"Connextion Info.vi"() -> ("Connected"=→"NT Connection":bool)  [unwired: 10 in, 1 out]
      }
      event "Test Tree": Value Change {
        # "Show appropriate\ncontrols"
        n164 = event-data() -> ("CtlRef"=w318:refnum<vi>, "NewVal"=w316:string)  [unwired: 1 in]
        n165 = call <vilib>:"WPI_UtilitiesGetTreeIOName.vi"("NewVal"=w316, "TreeControl in"=w318) -> ("I/O Name"=w319:string)  [unwired: 9 in]
        n166 = case shown="\"Camera\"" w319 {
          selector: w319 -> [_ w326 _ w348 w357 _]
          tunnel: w316 -> [_ _ w345 w347 _ w364]
          tunnel: cluster{string[]}[] [{["640x480", "320x240", "160x120"]}, {["Auto", "Fixed indoor", "Fixed outdoor 1", "Fixed outdoor 2", "Fixed fluorescent 1", "Fixed fluorescent 2", "Hold current"]}, {["Auto", "Flicker-free 50 Hz", "Flicker-free 60 Hz", "Hold current"]}, {["None", "Prioritize frame rate", "Prioritize image quality"]}, {["Monochrome", "Color"]}] -> [_ _ _ _ _ w363]
          frame Default {
            w321 = FALSE ("Visible")
            w320 = FALSE ("Visible")
            n167 = property on="Motor" class="Clust (strict)"("Visible"=w320) -> ()  [unwired: 2 in, 2 out]
            n168 = property on="Test Ring" class="Ring (strict)"("Visible"=w320) -> ()  [unwired: 2 in, 2 out]
            n169 = property on="Rev/Fwd" class="Clust (strict)"("Visible"=w321) -> ()  [unwired: 2 in, 2 out]
            n170 = property on="On/Off" class="Bool (strict)"("Visible"=w321) -> ()  [unwired: 2 in, 2 out]
            n171 = property on="Test Slider" class="Slide (strict)"("Visible"=w321) -> ()  [unwired: 2 in, 2 out]
          }
          frame "Analog Out", "Motor", "PWM" {
            w327 = FALSE ("Visible")
            n172 = case shown="\"Analog Out\"" w326 {
              tunnel: [1.0 ("Value") -1.0 ("Value") 0.0 ("Value")] -> w325
              tunnel: [255.0 ("Value") 1.0 ("Value") 5.0 ("Value")] -> w324
              tunnel: [128.0 ("Value") 0.0 ("Value") 0.0 ("Value")] -> w323
              tunnel: [64.0 ("Value") 0.5 ("Value") 1.0 ("Value")] -> w322
              frame "PWM" {
              }
              frame "Motor", Default {
              }
              frame "Analog Out" {
              }
            }
            n173 = property on="Motor" class="Clust (strict)"("Visible"=TRUE) -> ()  [unwired: 2 in, 2 out]
            n174 = property on="Value" class="Slide (strict)"("Value"=w323, "Scale.Minimum"=w325, "Scale.Maximum"=w324, "Scale.Increment"=w322) -> ()  [unwired: 2 in, 2 out]
            n175 = property on="On/Off" class="Bool (strict)"("Visible"=w327) -> ()  [unwired: 2 in, 2 out]
            n176 = property on="Test Slider" class="Slide (strict)"("Visible"=w327) -> ()  [unwired: 2 in, 2 out]
            n177 = property on="Test Ring" class="Ring (strict)"("Visible"=w327) -> ()  [unwired: 2 in, 2 out]
            n178 = property on="Rev/Fwd" class="Clust (strict)"("Visible"=w327) -> ()  [unwired: 2 in, 2 out]
          }
          frame "Servo" {
            w343 = FALSE ("Visible")
            n179 = call <vilib>:"NT Read Number.vi"("Name"=w345) -> ("Numeric"=w344:dbl)  [unwired: 9 in, 1 out]
            n180 = property on="Test Slider" class="Slide (strict)"("Visible"=TRUE, "Scale.Maximum"=170.0 ("Scale.Range:Maximum")) -> ()  [unwired: 2 in, 2 out]
            n181 = local write "Test Slider"(w344) -> ()
            n182 = property on="Motor" class="Clust (strict)"("Visible"=w343) -> ()  [unwired: 2 in, 2 out]
            n183 = property on="Rev/Fwd" class="Clust (strict)"("Visible"=w343) -> ()  [unwired: 2 in, 2 out]
            n184 = property on="On/Off" class="Bool (strict)"("Visible"=w343) -> ()  [unwired: 2 in, 2 out]
            n185 = property on="Test Ring" class="Ring (strict)"("Visible"=w343) -> ()  [unwired: 2 in, 2 out]
          }
          frame "Relay", "Solenoid" {
            w346 = FALSE ("Visible")
            n186 = property on="Motor" class="Clust (strict)"("Visible"=w346) -> ()  [unwired: 2 in, 2 out]
            n187 = property on="Test Slider" class="Slide (strict)"("Visible"=w346) -> ()  [unwired: 2 in, 2 out]
            n188 = Search and Replace String(input string=w347, search string="/Value  **", replace string="/Direction") -> (result string=w353:string)  [unwired: 5 in, 3 out]
            n189 = property on="Test Ring" class="Ring (strict)"("Visible"=w346) -> ()  [unwired: 2 in, 2 out]
            n190 = call <vilib>:"NT Read String.vi"("Name"=w353) -> ("String"=w351:string)  [unwired: 9 in, 1 out]
            n191 = Equal?(x="Both directions", y=w351) -> (x = y?=w349:bool)
            n192 = Not(x=w349) -> (.not. x?=w350:bool)
            n193 = property on="Rev/Fwd" class="Clust (strict)"("Visible"=w349) -> ()  [unwired: 2 in, 2 out]
            n194 = property on="On/Off" class="Bool (strict)"("Visible"=w350, "Caption.Text"=w348) -> ()  [unwired: 2 in, 2 out]
          }
          frame "Compressor", "Digital Out" {
            w356 = FALSE ("Visible")
            # "Get direction and finish"
            n195 = property on="Motor" class="Clust (strict)"("Visible"=w356) -> ()  [unwired: 2 in, 2 out]
            n196 = property on="Test Slider" class="Slide (strict)"("Visible"=w356) -> ()  [unwired: 2 in, 2 out]
            n197 = property on="Test Ring" class="Ring (strict)"("Visible"=w356) -> ()  [unwired: 2 in, 2 out]
            n198 = property on="On/Off" class="Bool (strict)"("Visible"=TRUE, "Caption.Text"=w357) -> ()  [unwired: 2 in, 2 out]
            n199 = property on="Rev/Fwd" class="Clust (strict)"("Visible"=FALSE) -> ()  [unwired: 2 in, 2 out]
          }
          frame "Camera" {
            n200 = call <vilib>:"Get Last Path Segment.vi"("String in"=w364) -> ("String out"=w365:string)  [unwired: 10 in]
            n201 = property on="On/Off" class="Bool (strict)"("Visible"=FALSE) -> ()  [unwired: 2 in, 2 out]
            n202 = property on="Motor" class="Clust (strict)"("Visible"=FALSE) -> ()  [unwired: 2 in, 2 out]
            n203 = property on="Rev/Fwd" class="Clust (strict)"("Visible"=FALSE) -> ()  [unwired: 2 in, 2 out]
            n204 = case shown="\"White Balance  **\"" w365 {
              tunnel: w364 -> [w371 w380 w389 w398 w407 _ w413]
              tunnel: w363 -> [w369 w377 w386 w395 w404 _ _]
              frame "Size  **" {
                n205 = Index Array(array=w369) -> (element=w368:cluster{string[]})  [unwired: 1 in]
                n206 = call <vilib>:"NT Read String.vi"("Name"=w371) -> ("String"=w370:string)  [unwired: 9 in, 1 out]
                n207 = Unbundle(w368) -> (w366:string[])
                n208 = Match First String(2:w366, 3:w370) -> (0:w367:i32)  [unwired: 1 out]
                n209 = property on="Test Ring" class="Ring (strict)"("Value"=w367, "Strings []"=w366) -> ()  [unwired: 2 in, 2 out]
                n210 = property on="Test Ring" class="Ring (strict)"("Visible"=TRUE) -> ()  [unwired: 2 in, 2 out]
                n211 = property on="Test Slider" class="Slide (strict)"("Visible"=FALSE) -> ()  [unwired: 2 in, 2 out]
              }
              frame "White Balance  **" {
                n212 = Index Array(array=w377, index=1) -> (element=w378:cluster{string[]})
                n213 = call <vilib>:"NT Read String.vi"("Name"=w380) -> ("String"=w379:string)  [unwired: 9 in, 1 out]
                n214 = Unbundle(w378) -> (w375:string[])
                n215 = Match First String(2:w375, 3:w379) -> (0:w374:i32)  [unwired: 1 out]
                n216 = property on="Test Ring" class="Ring (strict)"("Value"=w374, "Strings []"=w375) -> ()  [unwired: 2 in, 2 out]
                n217 = property on="Test Ring" class="Ring (strict)"("Visible"=TRUE) -> ()  [unwired: 2 in, 2 out]
                n218 = property on="Test Slider" class="Slide (strict)"("Visible"=FALSE) -> ()  [unwired: 2 in, 2 out]
              }
              frame "Exposure  **" {
                n219 = Index Array(array=w386, index=2) -> (element=w387:cluster{string[]})
                n220 = call <vilib>:"NT Read String.vi"("Name"=w389) -> ("String"=w388:string)  [unwired: 9 in, 1 out]
                n221 = Unbundle(w387) -> (w383:string[])
                n222 = Match First String(2:w383, 3:w388) -> (0:w384:i32)  [unwired: 1 out]
                n223 = property on="Test Ring" class="Ring (strict)"("Value"=w384, "Strings []"=w383) -> ()  [unwired: 2 in, 2 out]
                n224 = property on="Test Ring" class="Ring (strict)"("Visible"=TRUE) -> ()  [unwired: 2 in, 2 out]
                n225 = property on="Test Slider" class="Slide (strict)"("Visible"=FALSE) -> ()  [unwired: 2 in, 2 out]
              }
              frame "Exposure Priority  **" {
                n226 = Index Array(array=w395, index=3) -> (element=w396:cluster{string[]})
                n227 = call <vilib>:"NT Read String.vi"("Name"=w398) -> ("String"=w397:string)  [unwired: 9 in, 1 out]
                n228 = Unbundle(w396) -> (w392:string[])
                n229 = Match First String(2:w392, 3:w397) -> (0:w393:i32)  [unwired: 1 out]
                n230 = property on="Test Ring" class="Ring (strict)"("Value"=w393, "Strings []"=w392) -> ()  [unwired: 2 in, 2 out]
                n231 = property on="Test Ring" class="Ring (strict)"("Visible"=TRUE) -> ()  [unwired: 2 in, 2 out]
                n232 = property on="Test Slider" class="Slide (strict)"("Visible"=FALSE) -> ()  [unwired: 2 in, 2 out]
              }
              frame "Color Enable  **" {
                n233 = Index Array(array=w404, index=4) -> (element=w405:cluster{string[]})
                n234 = call <vilib>:"NT Read String.vi"("Name"=w407) -> ("String"=w406:string)  [unwired: 9 in, 1 out]
                n235 = Unbundle(w405) -> (w401:string[])
                n236 = Match First String(2:w401, 3:w406) -> (0:w402:i32)  [unwired: 1 out]
                n237 = property on="Test Ring" class="Ring (strict)"("Value"=w402, "Strings []"=w401) -> ()  [unwired: 2 in, 2 out]
                n238 = property on="Test Ring" class="Ring (strict)"("Visible"=TRUE) -> ()  [unwired: 2 in, 2 out]
                n239 = property on="Test Slider" class="Slide (strict)"("Visible"=FALSE) -> ()  [unwired: 2 in, 2 out]
              }
              frame Default {
                n240 = property on="Test Ring" class="Ring (strict)"("Visible"=FALSE) -> ()  [unwired: 2 in, 2 out]
                n241 = property on="Test Slider" class="Slide (strict)"("Visible"=FALSE) -> ()  [unwired: 2 in, 2 out]
              }
              frame "Brightness  **", "Color Level  **", "Compression  **", "FPS  **", "Sharpness  **" {
                n242 = call <vilib>:"NT Read Number.vi"("Name"=w413) -> ("Numeric"=w412:dbl)  [unwired: 9 in, 1 out]
                n243 = local write "Test Slider"(w412) -> ()
                n244 = property on="Test Slider" class="Slide (strict)"("Visible"=TRUE, "Scale.Maximum"=100.0 ("Scale.Range:Maximum")) -> ()  [unwired: 2 in, 2 out]
                n245 = property on="Test Ring" class="Ring (strict)"("Visible"=FALSE) -> ()  [unwired: 2 in, 2 out]
              }
            }
          }
        }
        n246 = property on="Progress" class="Clust (strict)"("Visible"=FALSE) -> ()  [unwired: 2 in, 2 out]
      }
      event "Test Name": Mouse Enter {
        # "Populate the ring with the list of tests"
        n247 = event-data() -> ()  [unwired: 1 in, 1 out]
        n248 = call <vilib>:"NT Read String Array.vi"("Name"="/TestMode/TestList") -> ("String Array"=w421:string[])  [unwired: 9 in, 1 out]
        n249 = Build Array (concatenate)("Select the test to run...", w421) -> (w420:string[])
        n250 = property on="Test Name" class="Ring (strict)"("Strings []"=w420) -> ()  [unwired: 2 in, 2 out]
      }
      event "Test Name": Value Change {
        w423 = FALSE ("Visible")
        # "Tell the robot the test name to run"
        n251 = event-data() -> ("NewVal"=w427:u16)  [unwired: 1 in]
        n252 = property on="Test Name" class="Ring (strict)"() -> ("Strings []"=w428:string[])  [unwired: 2 in, 2 out]
        n253 = local write "Progress"(T7 {"Test Progress"=0, "Test Progress Text"=""} ("Progress")) -> ()
        n254 = Index Array(array=w428, index=w427) -> (element=w426:string)
        n255 = call <vilib>:"NT Write String.vi"("String"=w426, "Name"="/TestMode/TestName") -> ()  [unwired: 9 in, 1 out]
        n256 = property on="Progress" class="Clust (strict)"("Visible"=TRUE) -> ()  [unwired: 2 in, 2 out]
        n257 = property on="Motor" class="Clust (strict)"("Visible"=w423) -> ()  [unwired: 2 in, 2 out]
        n258 = property on="Test Slider" class="Slide (strict)"("Visible"=w423) -> ()  [unwired: 2 in, 2 out]
        n259 = property on="On/Off" class="Bool (strict)"("Visible"=w423) -> ()  [unwired: 2 in, 2 out]
        n260 = property on="Rev/Fwd" class="Clust (strict)"("Visible"=w423) -> ()  [unwired: 2 in, 2 out]
        n261 = property on="Test Ring" class="Ring (strict)"("Visible"=w423) -> ()  [unwired: 2 in, 2 out]
      }
      event "Select Auto": Mouse Enter {
        # "Populate the combo box with the list of autonomous options"
        n262 = event-data() -> ()  [unwired: 1 in, 1 out]
        n263 = call <vilib>:"NT Read String Array.vi"("Name"="Auto List") -> ("String Array"=w430:string[])  [unwired: 9 in, 1 out]
        n264 = property on="Select Auto" class="CmbBox"("Strings[]"=w430) -> ()  [unwired: 2 in, 2 out]
      }
      event "Select Auto": Value Change {
        # "User modified the Auto Selection. Write to NT variable so robot knows."
        n265 = event-data() -> ("NewVal"=w433:string)  [unwired: 1 in]
        n266 = call <vilib>:"NT Write String.vi"("String"=w433, "Name"="Auto Selector") -> ()  [unwired: 9 in, 1 out]
      }
      event "Command Selection": Value Change {
        # "Get the params and show in table"
        n267 = event-data() -> ("NewVal"=w439:i32)  [unwired: 1 in]
        n268 = property on="Command Selection" class="MCListbox (strict)"() -> ("ItemNames"=w437:string[][])  [unwired: 2 in, 2 out]
        n269 = call <vilib>:"WPI_DashboardUpdate Command Params.vi"("NewVal"=w439, "Commands"=w437, "Param Tbl"=w438) -> ()  [unwired: 8 in, 1 out]
      }
      event "Execute Command": Value Change {
        # "Started one, Unique ID holds\nresponse"
        n270 = event-data() -> ()  [unwired: 1 in, 1 out]
        n271 = property on="Command Selection" class="MCListbox (strict)"() -> ("ItemNames"=w450:string[][])  [unwired: 2 in, 2 out]
        n272 = Index Array(array=w450, index (row)="Command Selection", index (col)=0) -> (element=w448:string)
        n273 = call <vilib>:"Invoke Commands.vi"("Command Params"="Command Params", "Function Name"=w448) -> ("Params"=w444:u8, "Started"=w443:bool)  [unwired: 7 in, 1 out]
        n274 = Array Subset(array="Command Params", length (row)=w444) -> (w445:string[][])  [unwired: 3 in]
        n275 = Select(t="Executing" ("Cmd Status"), s=w443, f="" ("Cmd Status")) -> (s? t:f=→"Cmd Status":string)
      }
      event "Command Selection": Double Click {
        n276 = event-data() -> ("Row"=w458:i32)  [unwired: 1 in]
        n277 = property on="Command Selection" class="MCListbox (strict)"() -> ("ItemNames"=w461:string[][])  [unwired: 2 in, 2 out]
        n278 = local read "Command Params"() -> (w457:string[][])
        n279 = Index Array(array=w461, index (row)=w458, index (col)=0) -> (element=w459:string)
        n280 = call <vilib>:"Invoke Commands.vi"("Command Params"=w457, "Function Name"=w459) -> ("Params"=w456:u8, "Started"=w451:bool)  [unwired: 7 in, 1 out]
        n281 = Array Subset(array=w457, length (row)=w456) -> (w455:string[][])  [unwired: 3 in]
        n282 = Select(t="Executing" ("Cmd Status"), s=w451, f="" ("Cmd Status")) -> (s? t:f=w452:string)
        n283 = local write "Cmd Status"(w452) -> ()
      }
      event "CheckList": Double Click {
        # "Shift clears all"
        # "Update symbols on the listbox"
        n284 = event-data() -> ("PlatMods.Shift"=w463:bool, "Row"=w465:i32)  [unwired: 1 in]
        n285 = case shown="True" w463 {
          tunnel: w465 -> [w469 _]
          tunnel: 1 -> [w468 _]
          frame False {
            n286 = property on="CheckList" class="LstBox (strict)"() -> ("Item Symbols"=w467:i32[])  [unwired: 2 in, 2 out]
            n287 = Replace Array Subset(array=w467, new element=w468, index=w469) -> (w466:i32[])
            n288 = property on="CheckList" class="LstBox (strict)"("Item Symbols"=w466) -> ()  [unwired: 2 in, 2 out]
          }
          frame True {
            w470 = 0 ("Top Row")
            n289 = property on="CheckList" class="LstBox (strict)"() -> ("Number of Rows"=w472:u32)  [unwired: 2 in, 2 out]
            n290 = Initialize Array(0, w472) -> (w471:i32[])
            n291 = property on="CheckList" class="LstBox (strict)"("Top Row"=w470, "Value"=w470, "Item Symbols"=w471) -> ()  [unwired: 2 in, 2 out]
          }
        }
      }
      event "CheckList": Key Down {
        # "Update symbols on the listbox\nLeft and right keys check and uncheck"
        n292 = event-data() -> ("VKey"=w476:T25)  [unwired: 1 in]
        n293 = case shown="\"Left\", \"Right\"" w476 {
          selector: w476 -> [w481 _]
          tunnel: eventvkey."Left" ("VKey") -> [w479 _]
          frame "Left", "Right" {
            n294 = Equal?(x=w479, y=w481) -> (x = y?=w480:bool)
            n295 = Select(t=0, s=w480, f=1) -> (s? t:f=w482:i32)
            n296 = property on="CheckList" class="LstBox (strict)"() -> ("Item Symbols"=w485:i32[])  [unwired: 2 in, 2 out]
            n297 = Replace Array Subset(array=w485, new element=w482, index="CheckList") -> (w484:i32[])
            n298 = property on="CheckList" class="LstBox (strict)"("Item Symbols"=w484) -> ()  [unwired: 2 in, 2 out]
          }
          frame Default {
          }
        }
      }
      event "Motor.Enable": Value Change {
        # "When the test mode otor enable helper is set, update that\ntree row item's value"
        n299 = event-data() -> ("NewVal"=w491:bool)  [unwired: 1 in]
        n300 = Unbundle("Motor") -> ("Value"=w490:dbl)  [unwired: 1 out]
        n301 = Select(t=w490, s=w491, f=0.0) -> (s? t:f=w488:dbl)
        n302 = call <vilib>:"NT Write Number.vi"("Numeric"=w488, "Name"=w487) -> ()  [unwired: 9 in, 1 out]
      }
      event "Test Slider": Value Change {
        # "When the test mode slider helper is set, update that\ntree row item's value"
        n303 = event-data() -> ("NewVal"=w494:dbl)  [unwired: 1 in]
        n304 = call <vilib>:"NT Write Number.vi"("Numeric"=w494, "Name"=w495) -> ()  [unwired: 9 in, 1 out]
      }
      event "On/Off": Value Change {
        # "When the test mode on/off helper value is set, update that\ntree row item's value"
        n305 = event-data() -> ("NewVal"=w499:bool)  [unwired: 1 in]
        n306 = Boolean To (0,1)(Boolean=w499) -> (0, 1=w498:i16)
        n307 = call <vilib>:"NT Write Number.vi"("Numeric"=w498, "Name"=w497) -> ()  [unwired: 9 in, 1 out]
      }
      event "Rev/Fwd": Value Change {
        # "When the test mode helper value for relays is set, update that\ntree row item's value"
        n308 = event-data() -> ("NewVal.Forward"=w507:bool, "NewVal.Reverse"=w506:bool)  [unwired: 1 in]
        n309 = Boolean To (0,1)(Boolean=w507) -> (0, 1=w503:i16)
        n310 = Boolean To (0,1)(Boolean=w506) -> (0, 1=w505:i16)
        n311 = Negate(x=w505) -> (-x=w504:i16)
        n312 = Add(x=w503, y=w504) -> (x+y=w502:i16)
        n313 = call <vilib>:"NT Write Number.vi"("Numeric"=w502, "Name"=w501) -> ()  [unwired: 9 in, 1 out]
      }
      event "Test Ring": Value Change {
        # "When a test mode helper value is selected from the ring,\nset the tree item's variable to the string value"
        n314 = event-data() -> ("NewVal"=w511:u16)  [unwired: 1 in]
        n315 = property on="Test Ring" class="Ring (strict)"() -> ("Strings []"=w512:string[])  [unwired: 2 in, 2 out]
        n316 = Index Array(array=w512, index=w511) -> (element=w510:string)
        n317 = call <vilib>:"NT Write String.vi"("String"=w510, "Name"=w509) -> ()  [unwired: 9 in, 1 out]
      }
      event "Rec Mode": Value Change {
        # "Update globals for recording mode and path to read log from.\nClear when logging and let NetworkTables set path for vision to\nuse."
        n318 = event-data() -> ("NewVal"=w523:enum32{"Stop", "Record", "Playback"})  [unwired: 1 in]
        n319 = global write "WPI_DashboardLogging Global.vi" "Logging Filename"(path "") -> ()
        n320 = global write "WPI_DashboardLogging Global.vi" "Recording"(w523) -> ()
        n321 = case shown="\"Playback\"" w523 {
          tunnel: w522 -> [_ w525 w534]
          tunnel: [_ _ w533] -> w520
          tunnel: [_ _ w532] -> _
          tunnel: w518 -> [_ _ w530]
          tunnel: cluster{i32, i32} {-250, 170} -> [_ _ w529]
          tunnel: [_ _ T26 {"Image Size"=TRUE, "Image Type"=TRUE, "Pixel Value"=TRUE, "ROI Information"=TRUE, "Zoom Factor"=FALSE} ("Image Information Shown:All Elements")] -> w516
          tunnel: [_ _ TRUE ("Zoom Factor")] -> w515
          tunnel: w514 -> [_ _ w526]
          frame Default {
          }
          frame "Stop", "Record" {
            # "Place Window too"
            n322 = invoke class="VI" method="FP.Close"(reference=w525) -> (reference out=w524:refnum<vi>)  [unwired: 2 in, 2 out]
            n323 = invoke class="VI" method="Abort VI"(reference=w524) -> ()  [unwired: 2 in, 3 out]
          }
          frame "Playback" {
            n324 = call "Open Playback Panel.vi"("Offset"=w529, "DB VI Ref"=w530, "Playback in"=w534) -> ("Playback out"=w531:refnum<vi>)  [unwired: 8 in]
            n325 = register-events(w531, w526) -> (reference out=w533:refnum<event-registration>, error out=w532:errorcluster)  [unwired: 2 in]
          }
        }
        n326 = property on="Camera Image" class="ImageControl"("Image Information Shown"=w516, "Image Information Visible"=w515) -> ()  [unwired: 2 in, 2 out]
        n327 = call <vilib>:"WPI_DashboardNT Log FieldName Cache.vi"("Operation"=enum16{"Lookup/Add", "Index", "Clear"}."Clear") -> ()  [unwired: 8 in, 3 out]
      }
      event Panel Close {
        w536 = enum32{"Stop", "Record", "Playback"}."Stop" ("Rec Mode")
        # "Playback window has been closed, abort"
        n328 = event-data() -> ()  [unwired: 1 in, 4 out]
        n329 = local write "Rec Mode"(w536) -> ()
        n330 = global write "WPI_DashboardLogging Global.vi" "Recording"(w536) -> ()
      }
      event Panel Close {
        # "Abort playback window and ourself"
        n331 = event-data() -> ()  [unwired: 1 in, 4 out]
        n332 = invoke class="VI" method="FP.Close"(reference=w540) -> (reference out=w539:refnum<vi>)  [unwired: 2 in, 2 out]
        n333 = invoke class="VI" method="Abort VI"(reference=w539) -> (error out=w538:errorcluster)  [unwired: 2 in, 2 out]
        n334 = invoke class="VI" method="Abort VI"(error in=w538) -> ()  [unwired: 2 in, 3 out]
      }
      event User Event {
        n335 = event-data() -> ("IDs"=w547:cluster{"RPC field ID":u16, "Unique ID":u16}, "String"=w546:string)  [unwired: 1 in]
        n336 = Bundle("IDs"=w547, "String"=w546) -> (w545:T11)  [unwired: 1 in]
        n337 = call <vilib>:"Retrieve RPC Response.vi"("RPC Response"=w545) -> ("Output"=w543:string[][])  [unwired: 10 in]
        n338 = Build Array (concatenate)(w541, w543) -> (w542:string[][])
        n339 = local write "Command Params"(w542) -> ()
        n340 = local write "Cmd Status"("" ("Cmd Status")) -> ()
      }
      event "Tree": Double Click {
        n341 = event-data() -> ("PlatMods"=w551:T29, "Tag"=w550:string)  [unwired: 1 in]
        n342 = Unbundle(w551) -> ("Shift"=w549:bool)  [unwired: 4 out]
        n343 = Not(x=w549) -> (.not. x?=w548:bool)
        n344 = call <vilib>:"NT Update Persistence.vi"("Persistence"=w548, "Name"=w550) -> ()  [unwired: 9 in, 1 out]
      }
    }
  }
  n345 = while {
    tunnel: w64 -> [w554]
    i -> [w557]
    stop <- FALSE stop-if-true
    n346 = Wait (ms)(milliseconds to wait=u32 100) -> ()  [unwired: 1 out]
    n347 = case shown="\"Playback\"" "Rec Mode" {
      tunnel: w557 -> [_ _ w572]
      tunnel: [u32 2829099 ("Base Color") u32 11141120 ("Target Color") w561] -> w553
      frame "Stop", Default {
        # "Reset the color, extra updates don't cost much"
      }
      frame "Record" {
      }
      frame "Playback" {
        # "Playback"
        n348 = Quotient & Remainder(x=w572, y=u32 50 ("milliseconds to wait")) -> (x-y*floor(x/y)=w568:u32)  [unwired: 1 out]
        n349 = Divide(x=w568, y=u32 50 ("milliseconds to wait")) -> (x/y=w565:dbl)
        n350 = Multiply(x=6.283185307179586, y=w565) -> (x*y=w570:dbl)
        n351 = Sine(x=w570) -> (sin(x)=w569:dbl)
        n352 = Absolute Value(x=w569) -> (abs(x)=w562:dbl)
        n353 = call "Interpolate RGB Color.vi"("Proportion"=w562, "Target Color"=u32 30976, "Base Color"=u32 2829099) -> ("Result Color"=w561:u32)  [unwired: 8 in]
      }
    }
    n354 = property class="Pane"(reference=w554, "PaneColor"=w553) -> ()  [unwired: 1 in, 2 out]
  }
  n355 = local write "Dashboard Tab"(T2."Swerve" ("Dashboard Tab")) -> ()
  n356 = property on="On/Off" class="Bool (strict)"("Visible"=w33) -> ()  [unwired: 2 in, 2 out]
  n357 = property on="Motor" class="Clust (strict)"("Visible"=w33) -> ()  [unwired: 2 in, 2 out]
  n358 = property on="Progress" class="Clust (strict)"("Visible"=w33) -> ()  [unwired: 2 in, 2 out]
  n359 = property on="Test Ring" class="Ring (strict)"("Visible"=w33) -> ()  [unwired: 2 in, 2 out]
  n360 = property on="Rev/Fwd" class="Clust (strict)"("Visible"=w33) -> ()  [unwired: 2 in, 2 out]
  n361 = while {
    tunnel: u16 1741 ("timeout ms (25000)") -> [w574]
    stop <- FALSE stop-if-true
    n362 = TCP Create Listener(10:w574) -> (0:w573:errorcluster, 3:w575:refnum<k5>)  [unwired: 4 in, 1 out]
    n363 = case shown="No Error" w573 {
      selector: w573 -> [w577 _]
      tunnel: w575 -> [w578 _]
      frame No Error {
        n364 = while {
          tunnel: w578 -> [w581]
          tunnel: w577 -> [w580]
          stop <- FALSE stop-if-true
          n365 = TCP Wait On Listener(8:w580, 11:w581) -> (0:w582:errorcluster, 4:w583:refnum<k5>)  [unwired: 2 in, 3 out]
          n366 = local write "TCP"(w583) -> ()
          n367 = case shown="No Error" w582 {
            frame No Error {
            }
            frame Error {
              n368 = Wait (ms)(milliseconds to wait=u32 1000) -> ()  [unwired: 1 out]
            }
          }
        }
      }
      frame Error {
        n369 = Wait (ms)(milliseconds to wait=u32 1000) -> ()  [unwired: 1 out]
      }
    }
  }
  n370 = local write "Command Selection"(u16 0 ("milliseconds to wait")) -> ()
  n371 = local write "Command Params"(string[][] [] ("Command Params")) -> ()
  n372 = global write "WPI_DashboardLogging Global.vi" "Recording"(w58) -> ()
  n373 = local write "Rec Mode"(w58) -> ()
  n374 = call <vilib>:"NT Write String.vi"("String"="Select Auto", "Name"="Auto Selector") -> ()  [unwired: 9 in, 1 out]
